vi "Example_squares.vi"() -> ()   [LabVIEW 2019, in "VGA.lvlib"]
doc: "Use this VI to test Color over whole picture of monitor."
uses:
  VGA.lvlib
  <vilib>/Platform/TimedLoop/XDataNode/wakeup.ctl
  <vilib>/Platform/TimedLoop/XDataNode/XDNodeRunTimeDep.lvlib
  <vilib>/Platform/TimedLoop/XDataNode/nitl_modes.ctl
  <vilib>/Platform/TimedLoop/XDataNode/timing_clust.ctl
  <vilib>/platform/TimedLoop/XDataNode/XDataNode.xnode
  <vilib>/rvi/DataTransferAndStorage/Container/XNode/niFpgaContainer.xnode
  <vilib>/rvi/Memory/Memory_Emulation/nirvimemoryFastEmulation.vi
  <vilib>/rvi/Memory/Memory_Emulation/nirvimemoryEmulation.vi
panel:
  in  "Multiply":i32
  in  "Add":fxp<+,3,3>
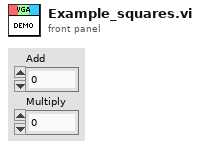
[diagram p1: front panel]
types:
  T1 = typedef "XDNodeRunTimeDep.lvlib/timing_clust.ctl" = cluster{"Expected End [f-1]":u64, "Actual End [f-1]":u64, "Finished Late? [f-1]":bool, "Expected End [i-1]":u64, "Actual End [i-1]":u64, "Finished Late? [i-1]":bool, "Expected Start [i]":u64, "Actual Start [i]":u64, "Expected Start [f]":u64, "Actual Start [f]":u64, "Source Name":string, "Structure Name":string, "Period":i64, "Deadline":i64, "Offset":i64, "Start":i64, "Priority":i32, "Timeout":i32, "Mode":T2, "Wakeup Reason":T3, "Error":errorcluster, "Source Type":string, "Secondary Source Type":string, "Global End Time":u64, "Global Start Time":u64, "Frame Duration":u64, "Iteration Duration":u64, "Assigned CPU":i32, "I/O Scan Engine Mode":u32}
  T2 = typedef "XDNodeRunTimeDep.lvlib/nitl_modes.ctl" = enum32{"No Change", "Process missed periods, maintain original phase", "Discard missed periods, maintain original phase", "Process missed periods, ignore original phase", "Discard missed periods, ignore original phase"}
  T3 = typedef "XDNodeRunTimeDep.lvlib/wakeup.ctl" = enum32{"Normal", "Aborted", "Asynchronous wakeup", "Timing source error", "Timed loop error", "Timeout"}
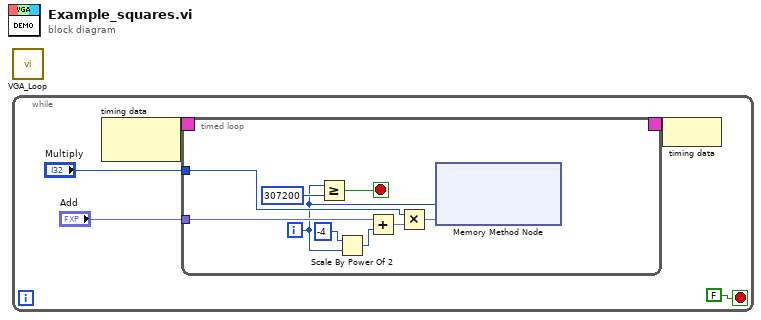
[diagram p0: block diagram]
diagram:
  n1 = call "VGA_Loop.vi"() -> ()  [unwired: 12 in]
  n2 = while {
    stop <- FALSE stop-if-true
    n3 = node-c288() -> (w5:T1)  [unwired: 1 in]
    n4 = timed-loop {
      timing: w5 -> [_]
      timing-out: [_] -> w4
      tunnel: "Multiply" -> [w10]
      tunnel: "Add" -> [w9]
      i -> [w7]
      stop <- w6 stop-if-true
      n5 = Greater Or Equal?(x=w7, y=307200) -> (x >= y?=w6:bool)
      n6 = Scale By Power Of 2(n=i16 -4, x=w7) -> (x*2^n=w12:i32)
      n7 = Add(x=w9, y=w12) -> (x+y=w11:fxp<+,3,3>)
      n8 = Multiply(x=w10, y=w11) -> (x*y=w8:fxp<+,3,3>)
      n9 = xnode ("Memory Method Node")("Address"=w7, "Data"=w8) -> ()  [unwired: 1 in, 1 out]
    }
    n10 = node-c288(w4) -> ()
  }
